vi "INST GLOBAL.vi"() -> ()   [LabVIEW 2018]
panel:
  out "Use_PS2":bool
  out "Use_PS1":bool
  out "Use PS2:4":bool[](array[boolean])
  out "Use PS2-2":bool
  out "Use PS2-1":bool
  out "Use PS1:4":bool[](array[boolean])
  out "Use PS1-4":bool
  out "Use PS1-3":bool
  out "Use PS1-2":bool
  out "Use PS1-1":bool
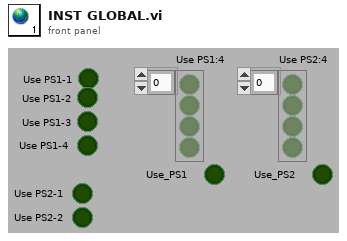
[diagram p1: front panel]
diagram:
